vi "Periodic Tasks.vi"(8 "error in":errorcluster) -> ()   [LabVIEW 2023]
doc: "This VI runs in parallel to other tasks. It can contain as many user-defined periodic loops as you need. These can carry out PID or other sorts of timed response."
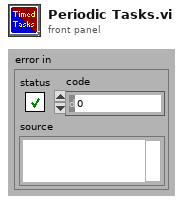
[diagram p1: front panel]
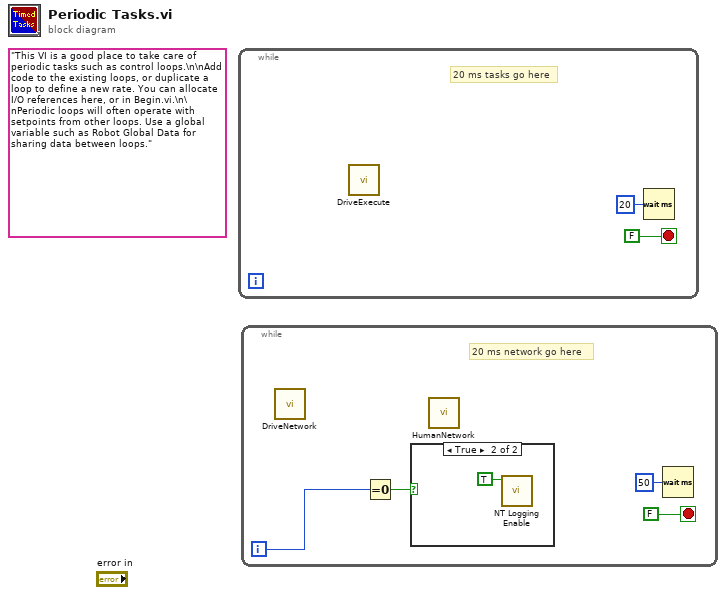
[diagram p0: block diagram]
diagram:
  (unwired) "This VI is a good place to take care of periodic tasks such as control loops.\n\nAdd code to the existing loops, or duplicate a loop to define a new rate. You can allocate I/O references here, or in Begin.vi.\n\nPeriodic loops will often operate with setpoints from other loops. Use a global variable such as Robot Global Data for sharing data between loops."
  n1 = while {
    stop <- FALSE stop-if-true
    # "20 ms tasks go here"
    n2 = call "DriveExecute.vi"() -> ()  [unwired: 11 in, 1 out]
    n3 = Wait (ms)(milliseconds to wait=u32 20) -> ()  [unwired: 1 out]
  }
  n4 = while {
    i -> [w4]
    stop <- FALSE stop-if-true
    # "20 ms network go here"
    n5 = call "DriveNetwork.vi"() -> ()  [unwired: 11 in, 1 out]
    n6 = Equal To 0?(x=w4) -> (x = 0?=w3:bool)
    n7 = case shown="True" w3 {
      frame False {
      }
      frame True {
        n8 = call <vilib>:"NT Logging Enable.vi"("Enable"=TRUE) -> ()  [unwired: 11 in]
      }
    }
    n9 = call "HumanNetwork.vi"() -> ()  [unwired: 11 in, 1 out]
    n10 = Wait (ms)(milliseconds to wait=u32 50) -> ()  [unwired: 1 out]
  }
